vi "shooterValue.vi"() -> (3 "Interpolated value":dbl)   [LabVIEW 2023]
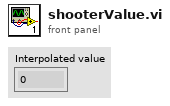
[diagram p1: front panel]
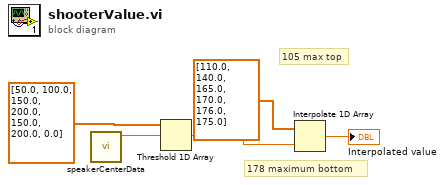
[diagram p0: block diagram]
diagram:
  # "105 max top"
  # "178 maximum bottom"
  n1 = call "speakerCenterData.vi"() -> ("DistanceToTarget (Inch)"=w2:dbl)  [unwired: 7 in, 3 out]
  n2 = Threshold 1D Array(2:w2, 3:dbl[] [50.0, 100.0, 150.0, 200.0, 150.0, 200.0, 0.0] ("array of numbers or points")) -> (0:w4:dbl)  [unwired: 1 in]
  n3 = Interpolate 1D Array(1:w4, 2:dbl[] [110.0, 140.0, 165.0, 170.0, 176.0, 175.0] ("array of numbers or points")) -> (0:→"Interpolated value":dbl)
